vi "矩形中心点（TB）.vi"(11 "矩形":T1) -> (3 "中心点":cluster{"x":i16, "y":i16})   [LabVIEW 2012]
uses:
  RectTB.ctl
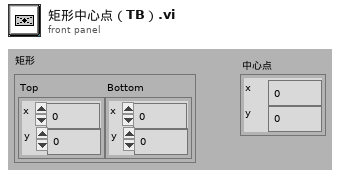
[diagram p1: front panel]
types:
  T1 = typedef "RectTB.ctl" = cluster{"Top":cluster{"x":i16, "y":i16}, "Bottom":cluster{"x":i16, "y":i16}}
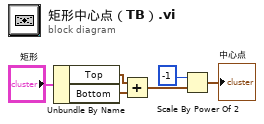
[diagram p0: block diagram]
diagram:
  n1 = Unbundle By Name("矩形") -> ("Top"=w5:cluster{"x":i16, "y":i16}, "Bottom"=w4:cluster{"x":i16, "y":i16})
  n2 = Add(x=w5, y=w4) -> (x+y=w3:cluster{"x":i16, "y":i16})
  n3 = Scale By Power Of 2(n=-1, x=w3) -> (x*2^n=→"中心点":cluster{"x":i16, "y":i16})
